vi "SimAdc Fetch Samples.vi"(8 "error in":errorcluster, 10 "max samples per fetch (1M)":i64=1000000, 11 "simadc in":T1) -> (0 "error out":errorcluster, 1 "done":bool, 2 "sample data":i32[][](array[numeric]), 3 "simadc out":T1, 4 "samples fetched":i64, 5 "scale factor [V]":dbl, 6 "smpl offset":i64, 7 "Ts [s]":dbl, 9 "time stamp [s]":dbl)   [LabVIEW 2020]
doc: "Fetches simulated samples from the ADC."
uses:
  SimAdc Config.ctl
  SimAdc Channel Cfg.ctl
  <vilib>/Analysis/baseanly.llb/Real A x B.vi
  <vilib>/Analysis/Matrix/Numeric/Conversions/Array To Matrix - RA.vi
  <vilib>/Analysis/Matrix/Numeric/Add/Add - RM,RM.vi
  <vilib>/Analysis/Matrix/Numeric/Conversions/Matrix To Array - RM.vi
  <vilib>/Analysis/Matrix/NI_Matrix.lvlib
  <vilib>/Analysis/NI_AALBase.lvlib
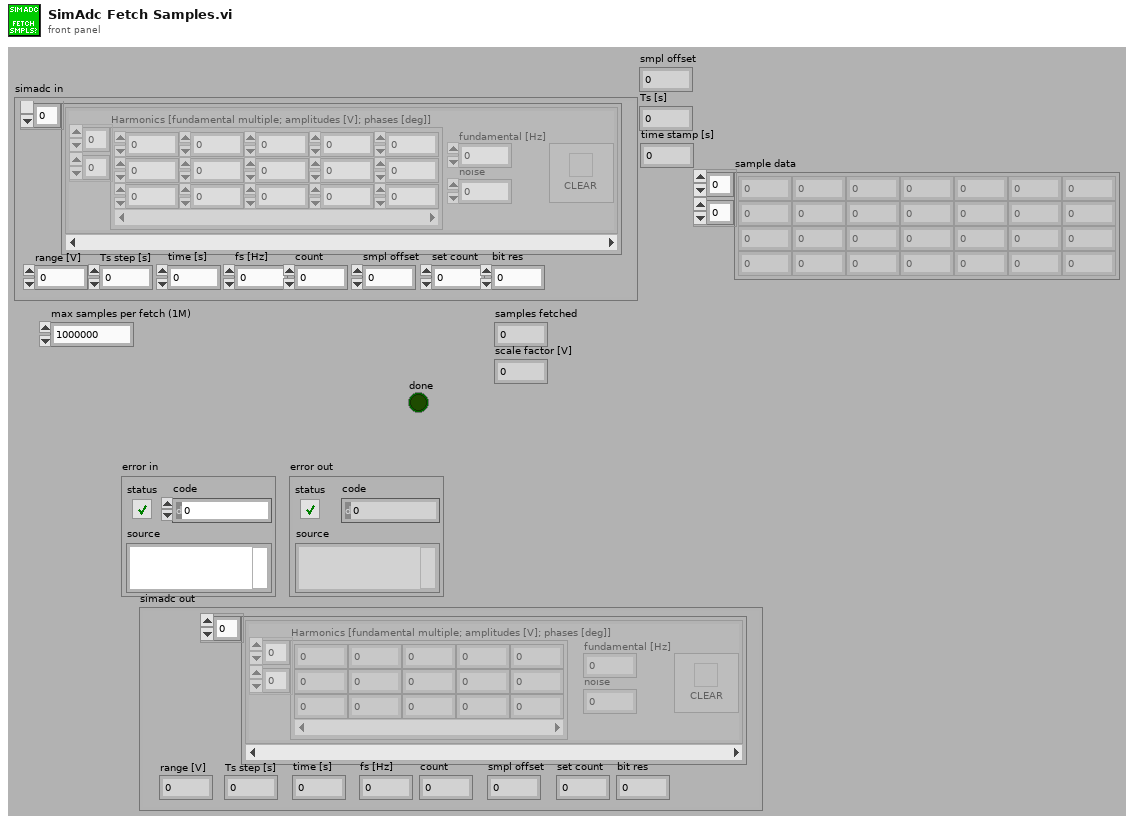
[diagram p1: front panel]
types:
  T1 = typedef "SimAdc Config.ctl" = cluster{"channels":T2[], "range [V]":dbl, "Ts step [s]":dbl, "time [s]":dbl, "fs [Hz]":dbl, "count":i64, "smpl offset":i64, "set count":i64, "bit res":i32}
  T2 = typedef "SimAdc Channel Cfg.ctl" = cluster{"harmonics":dbl[][], "btn clear":bool, "noise":dbl, "fundamental [Hz]":dbl}
  T3 = typedef "NI_Matrix.lvlib/RealMatrix.ctl" = dbl[][]
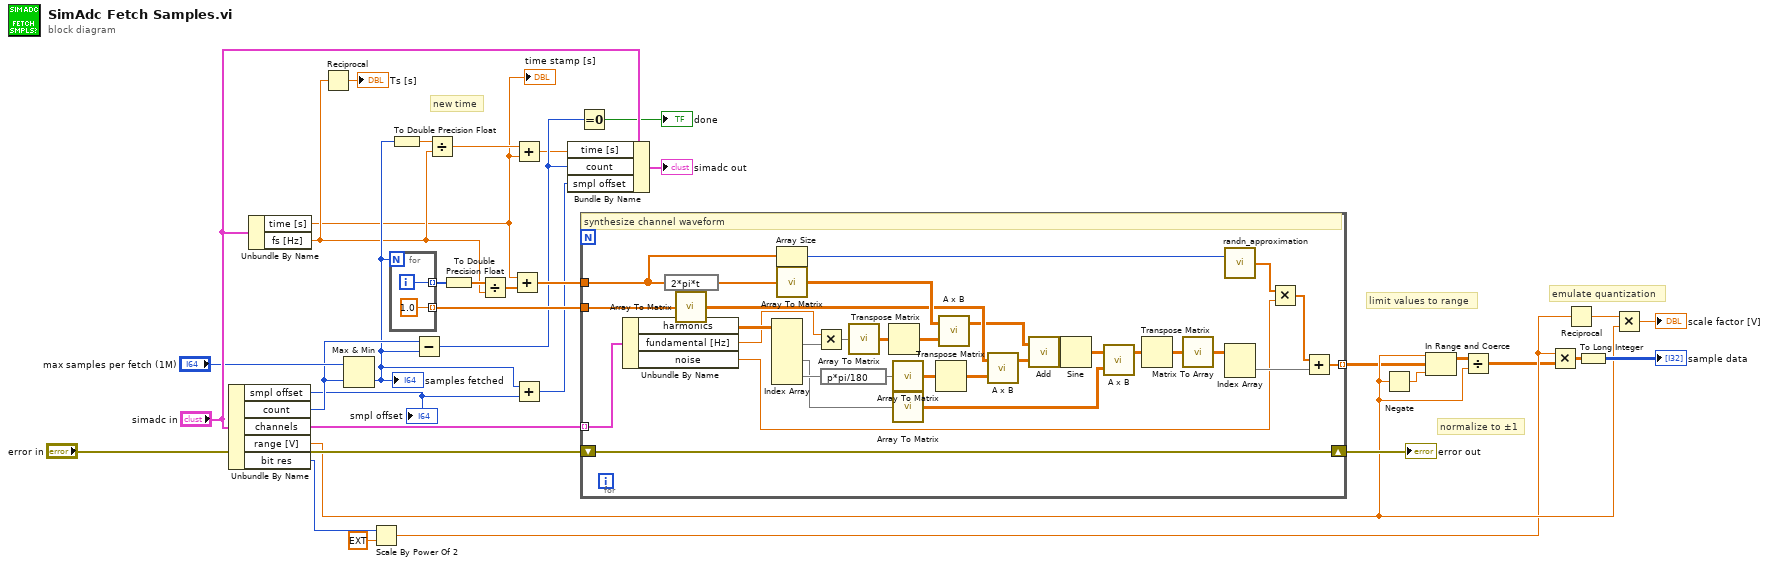
[diagram p0: block diagram]
diagram:
  # "emulate quantization"
  # "normalize to ±1"
  # "limit values to range"
  # "new time"
  n1 = Unbundle By Name("simadc in") -> ("smpl offset"=w19:i64, "count"=w24:i64, "channels"=w35:T2[], "range [V]"=w11:dbl, "bit res"=w9:i32)
  "smpl offset" <- w19
  n2 = Unbundle By Name("simadc in") -> ("time [s]"=w1:dbl, "fs [Hz]"=w16:dbl)
  "time stamp [s]" <- w1
  n3 = Reciprocal(x=w16) -> (1/x=→"Ts [s]":dbl)
  n4 = Max & Min(x="max samples per fetch (1M)", y=w24) -> (min(x,y)=w18:i64)  [unwired: 1 out]
  "samples fetched" <- w18
  n5 = Scale By Power Of 2(n=w9, x=ext 1.0) -> (x*2^n=w7:ext)
  n6 = for {
    N: w18 -> [_]
    tunnel: [w37] -> w31 mode=indexing
    tunnel: [1.0] -> w25 mode=indexing
    i -> [w37]
  }
  n7 = To Double Precision Float(number=w18) -> (double precision float=w28:dbl)
  n8 = Subtract(x=w24, y=w18) -> (x-y=w23:i64)
  n9 = Divide(x=w28, y=w16) -> (x/y=w3:dbl)
  n10 = To Double Precision Float(number=w31) -> (double precision float=w30:dbl[])
  n11 = Divide(x=w30, y=w16) -> (x/y=w29:dbl[])
  n12 = Add(x=w1, y=w29) -> (x+y=w27:dbl[])
  n13 = Add(x=w3, y=w1) -> (x+y=w2:dbl)
  n14 = Add(x=w18, y=w19) -> (x+y=w17:i64)
  n15 = Bundle By Name(cluster="simadc in", "time [s]"=w2, "count"=w23, "smpl offset"=w17) -> (→"simadc out":T1)
  n16 = Equal To 0?(x=w23) -> (x = 0?=→"done":bool)
  n17 = for {
    shift-right: [w69] -> w33
    shift-left: "error in" -> [w69]
    tunnel: w35 -> [w68] mode=indexing
    tunnel: w27 -> [w44]
    tunnel: w25 -> [w57]
    tunnel: [w41] -> w5 mode=indexing
    # "synthesize channel waveform"
    n18 = Unbundle By Name(w68) -> ("harmonics"=w67:dbl[][], "fundamental [Hz]"=w65:dbl, "noise"=w39:dbl)
    n19 = expression code="2*pi*t"(w44) -> (w62:dbl[])
    n20 = call-poly <vilib>:"Array To Matrix.vi"("Real 1D Array"=w57) -> ("Real Matrix (Column Vector)"=w55:T3)
    n21 = Index Array(array=w67) -> (element #1=w66:dbl[], element #2=w50:dbl[], element #3=w59:dbl[])  [unwired: 6 in]
    n22 = Array Size(array=w44) -> (size(s)=w43:i32)
    n23 = call-poly <vilib>:"Array To Matrix.vi"("Real 1D Array"=w62) -> ("Real Matrix (Column Vector)"=w60:T3)
    n24 = Multiply(x=w65, y=w66) -> (x*y=w64:dbl[])
    n25 = expression code="p*pi/180"(w59) -> (w58:dbl[])
    n26 = call-poly <vilib>:"Array To Matrix.vi"("Real 1D Array"=w64) -> ("Real Matrix (Column Vector)"=w63:T3)
    n27 = Transpose Matrix(1:w63) -> (0:w61:T3)
    n28 = call-poly <vilib>:"Array To Matrix.vi"("Real 1D Array"=w58) -> ("Real Matrix (Column Vector)"=w56:T3)
    n29 = call-poly <vilib>:"Array To Matrix.vi"("Real 1D Array"=w50) -> ("Real Matrix (Column Vector)"=w48:T3)
    n30 = Transpose Matrix(1:w56) -> (0:w54:T3)
    n31 = call-poly <vilib>:"A x B.vi"("B"=w61, "A"=w60) -> ("A x B"=w52:T3)  [unwired: 1 out]
    n32 = call-poly <vilib>:"A x B.vi"("B"=w54, "A"=w55) -> ("A x B"=w53:T3)  [unwired: 1 out]
    n33 = call-poly <vilib>:"Add.vi"("Real Matrix B"=w53, "Real Matrix A"=w52) -> ("A + B"=w51:T3)
    n34 = Sine(x=w51) -> (sin(x)=w49:T3)
    n35 = call-poly <vilib>:"A x B.vi"("B"=w48, "A"=w49) -> ("A x B"=w47:T3)  [unwired: 1 out]
    n36 = Transpose Matrix(1:w47) -> (0:w45:T3)
    n37 = call-poly <vilib>:"Matrix To Array.vi"("Real Matrix"=w45) -> ("Real 2D Array"=w46:dbl[][])
    n38 = call "randn_approximation.vi"("N"=w43) -> ("randn() vector"=w40:dbl[])  [unwired: 1 in]
    n39 = Index Array(array=w46) -> (element=w42:dbl[])  [unwired: 2 in]
    n40 = Multiply(x=w40, y=w39) -> (x*y=w38:dbl[])
    n41 = Add(x=w38, y=w42) -> (x+y=w41:dbl[])
  }
  "error out" <- w33
  n42 = Negate(x=w11) -> (-x=w13:dbl)
  n43 = In Range and Coerce(upper limit=w11, x=w5, lower limit=w13) -> (coerced(x)=w4:dbl[][])  [unwired: 1 out]
  n44 = Divide(x=w4, y=w11) -> (x/y=w6:dbl[][])
  n45 = Multiply(x=w7, y=w6) -> (x*y=w21:ext[][])
  n46 = Reciprocal(x=w7) -> (1/x=w12:ext)
  n47 = To Long Integer(number=w21) -> (32bit integer=→"sample data":i32[][])
  n48 = Multiply(x=w12, y=w11) -> (x*y=→"scale factor [V]":ext)
